vi "Control Type.vi"(11 "SequencedValves in":refnum<class "TriggerDelayControl.lvclass">) -> (2 "Valve Type":string)   [LabVIEW 2020, in "VolatusControl.lvlib" / "TriggerDelayControl.lvclass"]
uses:
  TriggerDelayControl.lvclass
  TriggerDelayControl.lvclass/TriggerDelayControl.ctl
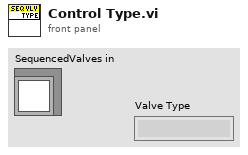
[diagram p1: front panel]
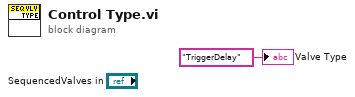
[diagram p0: block diagram]
diagram:
  "Valve Type" <- "TriggerDelay" ("Valve Type")
